vi "SCLB Initialize.vi"(8 "error in (no error)":errorcluster, 11 "MCLB_Template in":refnum<class "SCLB_Template.lvclass">) -> (0 "error out":errorcluster, 3 "MCLB_Template out":refnum<class "SCLB_Template.lvclass">)   [LabVIEW 2021, in "SCLB_Template.lvclass"]
uses:
  SCLB_Template.lvclass
  SCLB_Template.lvclass/SCLB_Template.ctl
  <userlib>/Control_Lib/SCLB_Lib/SCLB_Lib.lvclass
panel:
  in  "Config_CSV_FilePath":path
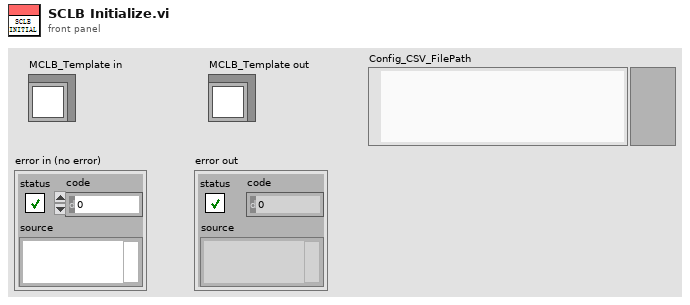
[diagram p1: front panel]
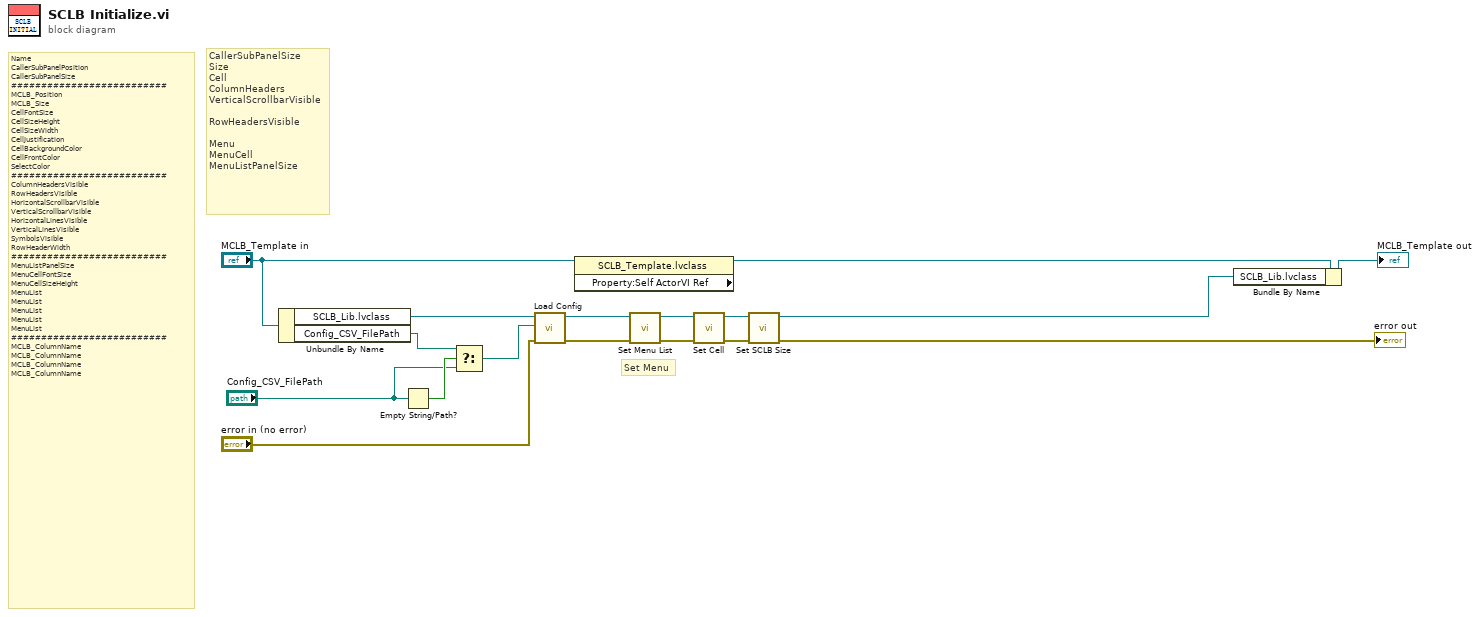
[diagram p0: block diagram]
diagram:
  # "Set Menu"
  # "Name\nCallerSubPanelPosition\nCallerSubPanelSize\n##########################\nMCLB_Position\nMCLB_Size\nCellFontSize\nCellSizeHeight\nCellSizeWidth\nCellJustification\nCellBackgroundColor\nCellFrontColor\nSelectColor\n##########################\nColumnHeadersVisible\nRowHeadersVisible\nHorizontalScrollbarVisible\nVerticalScrollbarVisible\nHorizontalLinesVisible\nVerticalLinesVisible\nSymbolsVisible\nRowHeaderWidth\n##########################\nMenuListPanelSize\nMenuCellFontSize\nMenuCellSizeHeight\nMenuList\nMenuList\nMenuList\nMenuList\nMenuList\n##########################\nMCLB_ColumnName\nMCLB_ColumnName\nMCLB_ColumnName\nMCLB_ColumnName"
  # "CallerSubPanelSize\nSize\nCell\nColumnHeaders\nVerticalScrollbarVisible\n\nRowHeadersVisible\n\nMenu\nMenuCell\nMenuListPanelSize"
  n1 = Unbundle By Name("MCLB_Template in") -> ("SCLB_Lib.lvclass"=w10:refnum<class "SCLB_Lib.lvclass">, "Config_CSV_FilePath"=w15:path)
  n2 = Empty String/Path?(string/path="Config_CSV_FilePath") -> (empty?=w17:bool)
  n3 = Select(t=w15, s=w17, f="Config_CSV_FilePath") -> (s? t:f=w14:path)
  n4 = call <userlib>:"Load Config.vi"("error in (no error)"="error in (no error)", "Config_CSV_FilePath"=w14, "SCLB_Lib in"=w10) -> ("error out"=w8:errorcluster, "SCLB_Lib out"=w9:refnum<class "SCLB_Lib.lvclass">)  [unwired: 7 in]
  n5 = property class="SCLB_Template.lvclass" props=["Property:Self ActorVI Ref"](reference="MCLB_Template in") -> (reference out=w1:refnum<class "SCLB_Template.lvclass">)  [unwired: 1 in, 2 out]
  n6 = call <userlib>:"Set Menu List.vi"("error in (no error)"=w8, "SCLB_Lib in"=w9) -> ("error out"=w6:errorcluster, "SCLB_Lib out"=w7:refnum<class "SCLB_Lib.lvclass">)  [unwired: 8 in]
  n7 = call <userlib>:"Set Cell.vi"("error in (no error)"=w6, "SCLB_Lib in"=w7) -> ("error out"=w4:errorcluster, "SCLB_Lib out"=w5:refnum<class "SCLB_Lib.lvclass">)  [unwired: 8 in]
  n8 = call <userlib>:"Set SCLB Size.vi"("error in (no error)"=w4, "MCLB_Lib in"=w5) -> ("error out"=→"error out":errorcluster, "MCLB_Lib out"=w3:refnum<class "SCLB_Lib.lvclass">)  [unwired: 7 in, 1 out]
  n9 = Bundle By Name(cluster=w1, "SCLB_Lib.lvclass"=w3) -> (→"MCLB_Template out":refnum<class "SCLB_Template.lvclass">)
